vi "testFlattenLengthToXML.vi"() -> ()   [LabVIEW 2012, in "UnitsAndXML.lvlib"]
uses:
  <userlib>/Common/UnitsAndXML/UnitsAndXML.lvlib
  <userlib>/Common/UnitsAndXML/FlattenItemWithUnitToXML/FlattenLengthToXML/LengthUnit.ctl
  <userlib>/Common/UnitsAndXML/FlattenItemWithUnitToXML/FlattenLengthToXML/typeMethods/flattenLengthToXML_Array.vi
  <userlib>/Common/UnitsAndXML/FlattenItemWithUnitToXML/FlattenLengthToXML/typeMethods/flattenLengthToXML_Scalar.vi
panel:
  out "error out":errorcluster
  in  "lengthUnitInXML":T1
  out "xmlStringArray":string
  out "xmlStringScalar":string
  in  "length":dbl[unit][](array[numeric])=[0.38099999999999995, 0.7619999999999999, 1.143, 1.5239999999999998]
  in  "length":dbl[unit]=0.38099999999999995
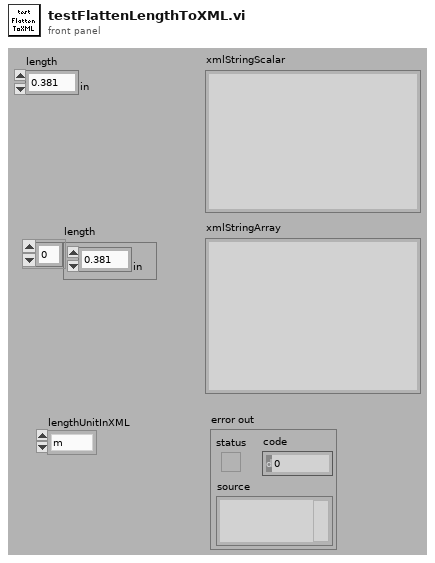
[diagram p1: front panel]
types:
  T1 = typedef "UnitsAndXML.lvlib/LengthUnit.ctl" = enum16{"m", "Angstrom", "AU", "chain", "cm", "cubit", "fathom", "fermi", "ft", "furlong", "hubble", "in", "ly", "mi", "mm", "rod", "um", "yd"}
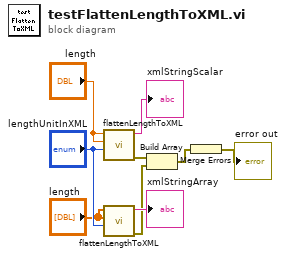
[diagram p0: block diagram]
diagram:
  n1 = call-poly <userlib>:"flattenLengthToXML.vi"("lengthUnitInXML"="lengthUnitInXML", "lengthAgain"="length", "length"="length") -> ("error out"=w6:errorcluster, "xmlString"=→"xmlStringScalar":string)  [unwired: 7 in]
  n2 = call-poly <userlib>:"flattenLengthToXML.vi"("lengthUnitInXML"="lengthUnitInXML", "timeAgain"="length", "length"="length") -> ("error out"=w1:errorcluster, "xmlString"=→"xmlStringArray":string)  [unwired: 7 in]
  n3 = Build Array(w6, w1) -> (w7:errorcluster[])
  n4 = Merge Errors(w7) -> (→"error out":errorcluster)
